vi "LPS22HH PPMU config.vi"(7 "channel list":string="VDD,VDDIO", 8 "error in":errorcluster, 9 "current limit range (A)":dbl=0.032 format="%#_13g", 10 "voltage level (V)":dbl=1.8 format="%#_13g", 11 "instrument handle":refnum<k15>) -> (0 "error out":errorcluster, 3 "instrument handle out":refnum<k15>)   [LabVIEW 2020, in "LPS22Demo.lvlib"]
uses:
  LPS22Demo.lvlib
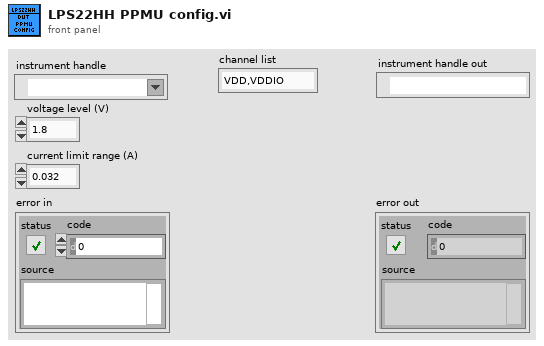
[diagram p1: front panel]
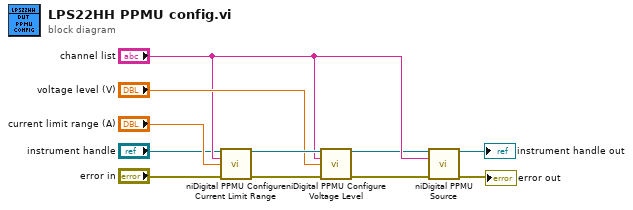
[diagram p0: block diagram]
diagram:
  n1 = call <instrlib>:"niDigital PPMU Configure Current Limit Range.vi"("instrument handle"="instrument handle", "channel list"="channel list", "current limit range (A)"="current limit range (A)", "error in"="error in") -> ("instrument handle out"=w9:refnum<k15>, "error out"=w10:errorcluster)  [unwired: 10 in]
  n2 = call <instrlib>:"niDigital PPMU Configure Voltage Level.vi"("instrument handle"=w9, "channel list"="channel list", "voltage level (V)"="voltage level (V)", "error in"=w10) -> ("instrument handle out"=w5:refnum<k15>, "error out"=w7:errorcluster)  [unwired: 10 in]
  n3 = call <instrlib>:"niDigital PPMU Source.vi"("instrument handle"=w5, "channel list"="channel list", "error in"=w7) -> ("instrument handle out"=→"instrument handle out":refnum<k15>, "error out"=→"error out":errorcluster)  [unwired: 11 in]
